vi "DataAcquisitionUpdate.vi"(6 "stop":bool) -> (4 "lineIndex":u32, 9 "linesPerUpdate":u16=1)   [LabVIEW 2016]
uses:
  controls/FPGAVIreferenceTypeDef.ctl
  controls/Enum.ctl
  <vilib>/Utility/error.llb/Error Cluster From Error Code.vi
  <vilib>/rvi/errors/niLvFpgaAdjustHostInterfaceError.vi
  <vilib>/rvi/interface/common/niFpgaWaitOnOcc.vi
  <vilib>/rvi/interface/nirviMethod/nirviMethod.xnode
  FPGA Bitfiles/lbniAFMControlle_flexRio_controllerFPGA.lvbitx
  controls/FPGAVIreferenceTypeDefScanEngine.ctl
  <vilib>/rvi/interface/nirviReadWriteControl/nirviReadWriteControl.xnode
  FPGA Bitfiles/lbniAFMControlle_scanControl_controllerFPGAPX_N4i+37z1gG8.lvbitx
  <vilib>/rvi/errors/niLvFpgaMergeErrorWithErrorCode.vi
  NiFpgaLv.dll
  <vilib>/FPGAPlugInAG/PXIe-7975R/niLvFpga_ConfigureFifo_PXIe-7975R.vi
  <vilib>/FPGAPlugInAG/PXIe-7975R/niLvFpga_StopFifo_PXIe-7975R.vi
panel:
  out "eltsRemaining":u32
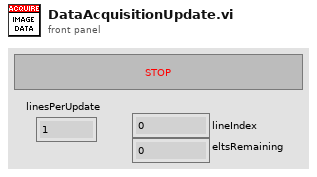
[diagram p1: front panel]
types:
  T1 = typedef "Enum.ctl" = enum16{"Init", "Read", "Write"}
  T2 = typedef "FPGAVIreferenceTypeDef.ctl" = refnum<k20>
  T3 = typedef "FPGAVIreferenceTypeDefScanEngine.ctl" = refnum<k20>
  T4 = typedef "ScanWaveform.ctl" = enum16{"Sine", "Triangle", "Rounded"}
  T5 = cluster{"slowWavePts":u16, "fastWavePts":u16, "slowWaveType":T4, "fastWaveType":T4, "slowRoundPts":u16, "fastRoundPts":u16, "singleDirectionScan":bool}
  T6 = cluster{"Width":dbl, "Height":dbl, "X Offset":dbl, "Y Offset":dbl, "Angle":dbl, "Pixels/Line":u16, "Lines":u16, "Time/Line":dbl, "Scan Rate":dbl}
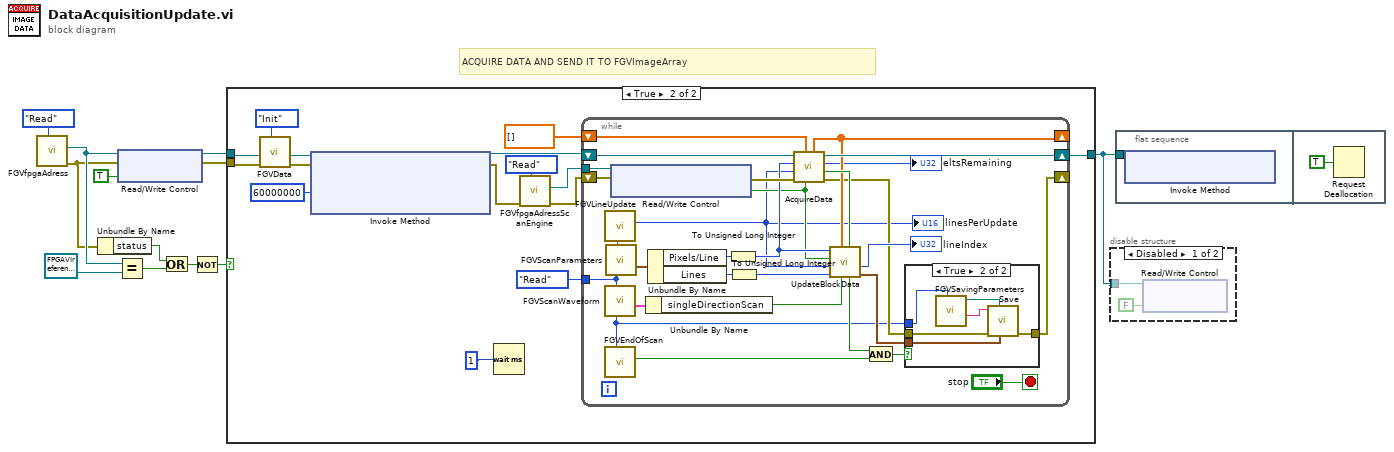
[diagram p0: block diagram]
diagram:
  # "ACQUIRE DATA AND SEND IT TO FGVImageArray"
  n1 = call "FGVfpgaAdress.vi"("Enum"=Enum."Read") -> ("error out"=w6:errorcluster, "FPGA VI Reference Out"=w7:T2)  [unwired: 5 in, 4 out]
  n2 = Unbundle By Name(w6) -> ("status"=w10:bool)
  n3 = Equal?(x=w7, y=T2 refnum ("FPGA VI Reference Out")) -> (x = y?=w9:bool)
  n4 = xnode "Read/Write Control"("FPGA VI Reference In"=w7, "error in"=w6, "hdt.o.enable"=TRUE) -> ("FPGA VI Reference Out"=w5:T2, "error out"=w4:errorcluster)
  n5 = Or(x=w10, y=w9) -> (x .or. y?=w11:bool)
  n6 = Not(x=w11) -> (.not. x?=w8:bool)
  n7 = case shown="True" w8 {
    tunnel: w5 -> [w13 w27]
    tunnel: w4 -> [_ w17]
    tunnel: [w13 w24] -> w2
    frame False {
    }
    frame True {
      n8 = call "FGVData.vi"("Enum"=Enum."Init", "error in"=w17) -> ("error out"=w16:errorcluster)  [unwired: 8 in, 1 out]
      n9 = xnode "Invoke Method"("FPGA VI Reference In"=w27, "error in"=w16, "Requested Depth"=u32 60000000) -> ("FPGA VI Reference Out"=w25:T2, "error out"=w18:errorcluster)  [unwired: 1 out]
      n10 = Wait (ms)(milliseconds to wait=u32 1) -> ()  [unwired: 1 out]
      n11 = call "FGVfpgaAdressScanEngine.vi"("Enum"=Enum."Read", "error in"=w18) -> ("error out"=w19:errorcluster, "FPGA.SEout"=w21:T3)  [unwired: 5 in, 3 out]
      n12 = while {
        tunnel: Enum."Read" ("Enum") -> [w29]
        shift-right: [w47] -> w24
        shift-left: w25 -> [w48]
        tunnel: w21 -> [w39]
        shift-right: [w37] -> _
        shift-left: sgl[] [] ("DataIn") -> [w38]
        shift-right: [w30] -> _
        shift-left: w19 -> [w35]
        stop <- "stop" stop-if-true
        n13 = call "FGVLineUpdate.vi"("Enum"=w29) -> ("LineUpdate"=w28:u16)  [unwired: 9 in, 1 out]
        "linesPerUpdate" <- w28
        n14 = call "FGVScanWaveform.vi"("Enum"=w29) -> ("scanWaveFormCtl Out"=w50:T5)  [unwired: 9 in, 1 out]
        n15 = call "FGVEndOfScan.vi"("Enum"=w29) -> ("autoSaveOut"=w46:bool)  [unwired: 9 in, 1 out]
        n16 = call "FGVScanParameters.vi"("Enum"=w29) -> ("Scan Parameters Out"=w51:T6)  [unwired: 9 in, 1 out]
        n17 = xnode "Read/Write Control"("FPGA VI Reference In"=w39, "error in"=w35) -> ("error out"=w54:errorcluster, "se.p.modes.se.p.enable"=w36:bool)  [unwired: 1 out]
        n18 = Unbundle By Name(w50) -> ("singleDirectionScan"=w49:bool)
        n19 = Unbundle By Name(w51) -> ("Pixels/Line"=w41:u16, "Lines"=w53:u16)
        n20 = To Unsigned Long Integer(number=w41) -> (unsigned 32bit integer=w40:u32)
        n21 = To Unsigned Long Integer(number=w53) -> (unsigned 32bit integer=w43:u32)
        n22 = call "AcquireData.vi"("ScanEnable"=w36, "DataIn"=w38, "error in"=w54, "linesPerUpdate"=w28, "Pixels/Line"=w40, "FPGA VI Reference In"=w48) -> ("error out"=w31:errorcluster, "BlockUpdate?"=w42:bool, "Elements Remaining"=→"eltsRemaining":u32, "FPGA VI Reference Out"=w47:T2, "DataOut"=w37:sgl[])  [unwired: 1 in]
        n23 = call "UpdateBlockData.vi"("BlockUpdate"=w42, "singleDirectionScan"=w49, "Data"=w37, "Lines"=w43, "linesPerUpdate"=w28, "ScanEnable?"=w36, "Pixels/Line"=w40) -> ("current time"=w33:timestamp, "LineIndex"=→"lineIndex":u32, "EndOfScan?"=w44:bool)  [unwired: 2 in]
        n24 = And(x=w44, y=w46) -> (x .and. y?=w45:bool)
        n25 = case shown="True" w45 {
          tunnel: w33 -> [_ w61]
          tunnel: w29 -> [_ w58]
          tunnel: w31 -> [w55 w57]
          tunnel: [w55 w56] -> w30
          frame False {
          }
          frame True {
            n26 = call "FGVSavingParameters.vi"("Enum"=w58) -> ("filenameOut"=w60:string, "pathOut"=w59:path)  [unwired: 7 in, 2 out]
            n27 = call "Save.vi"("current time"=w61, "base path"=w59, "error in"=w57, "Filename"=w60) -> ("error out"=w56:errorcluster)  [unwired: 6 in, 1 out]
          }
        }
      }
    }
  }
  n28 = disable-structure shown="Disabled" {
    disable-tunnel: w2 -> [w63 _]
    frame Disabled {
      n29 = xnode "Read/Write Control"("FPGA VI Reference In"=w63, "hdt.o.enable"=FALSE) -> ()  [unwired: 1 in, 2 out]
    }
    frame Enabled {
    }
  }
  n30 = flat-sequence {
    tunnel: w2 -> [w64]
    frame #0 {
      n31 = xnode "Invoke Method"("FPGA VI Reference In"=w64) -> ()  [unwired: 1 in, 2 out]
    }
    frame #1 {
      n32 = Request Deallocation(TRUE ("flag")) -> ()
    }
  }
